vi "XY Graph Get Plot Data Point near Point.vi"(8 "Error In":errorcluster, 9 "Point":cluster{"X":dbl, "Y":dbl}, 11 "Plot in":cluster{"X Array":dbl[], "Y Array":dbl[]}) -> (0 "Error Out":errorcluster, 1 "Point  Index":i32, 2 "Distance to Plot":dbl, 3 "Plot Data Point":cluster{"X":dbl, "Y":dbl})   [LabVIEW 2021, in "XY Graph Add-Ons.lvlib"]
uses:
  XY Graph Add-Ons.lvlib
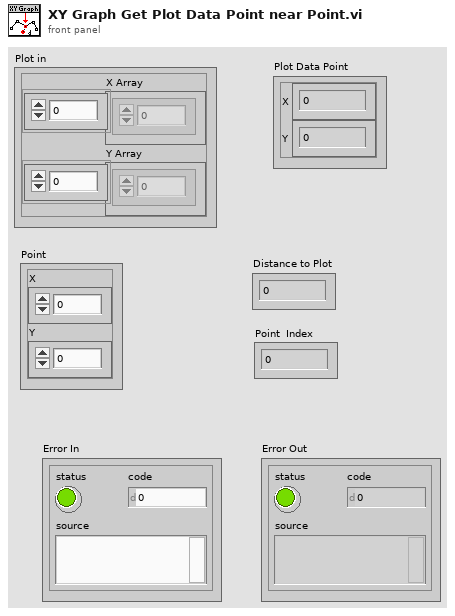
[diagram p1: front panel]
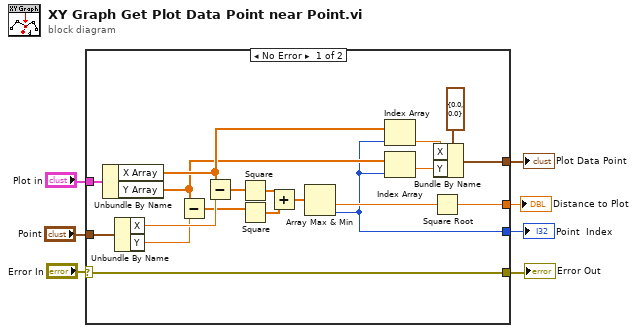
[diagram p0: block diagram]
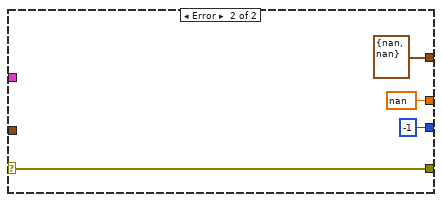
[diagram p2: hidden frame]
diagram:
  n1 = case shown="No Error" "Error In" {
    selector: "Error In" -> [w13 w30]
    tunnel: "Point" -> [w26 _]
    tunnel: [w17 nan] -> w6
    tunnel: "Plot in" -> [w14 _]
    tunnel: [w13 w30] -> w3
    tunnel: [w8 -1] -> w2
    tunnel: [w9 cluster{"X":dbl, "Y":dbl} {"X"=nan, "Y"=nan} ("Plot Data Point")] -> w1
    frame No Error {
      n2 = Unbundle By Name(w14) -> ("X Array"=w16:dbl[], "Y Array"=w15:dbl[])
      n3 = Unbundle By Name(w26) -> ("X"=w25:dbl, "Y"=w24:dbl)
      n4 = Subtract(x=w15, y=w24) -> (x-y=w22:dbl[])
      n5 = Subtract(x=w16, y=w25) -> (x-y=w23:dbl[])
      n6 = Square(x=w23) -> (x^2=w21:dbl[])
      n7 = Square(x=w22) -> (x^2=w20:dbl[])
      n8 = Add(x=w21, y=w20) -> (x+y=w19:dbl[])
      n9 = Array Max & Min(array=w19) -> (min value=w18:dbl, min index (indices)=w8:i32)  [unwired: 2 out]
      n10 = Index Array(array=w16, index=w8) -> (element=w11:dbl)
      n11 = Index Array(array=w15, index=w8) -> (element=w10:dbl)
      n12 = Square Root(x=w18) -> (sqrt(x)=w17:dbl)
      n13 = Bundle By Name(cluster=cluster{"X":dbl, "Y":dbl} {"X"=0.0, "Y"=0.0} ("Plot Data Point"), "X"=w11, "Y"=w10) -> (w9:cluster{"X":dbl, "Y":dbl})
    }
    frame Error {
    }
  }
  "Error Out" <- w3
  "Distance to Plot" <- w6
  "Point  Index" <- w2
  "Plot Data Point" <- w1
